vi "Snap To Grid.vi"(0 "Display State In":T1, 7 "Point In":T2) -> (8 "Point Out":cluster{"Horizontal":dbl, "Vertical":dbl})   [LabVIEW 2015, in "FSM Editor.xctl"]
uses:
  FSM Editor.xctl
  <vilib>/Utility/miscctls.llb/LVPoint32TypeDef.ctl
  State.vi
  Classes/FSM.Port/FSM.Port.lvclass
  Drag Mode.ctl
  Events.ctl
  NodeAdded.ctl
  NodeSelected.ctl
  EdgeEventData.ctl
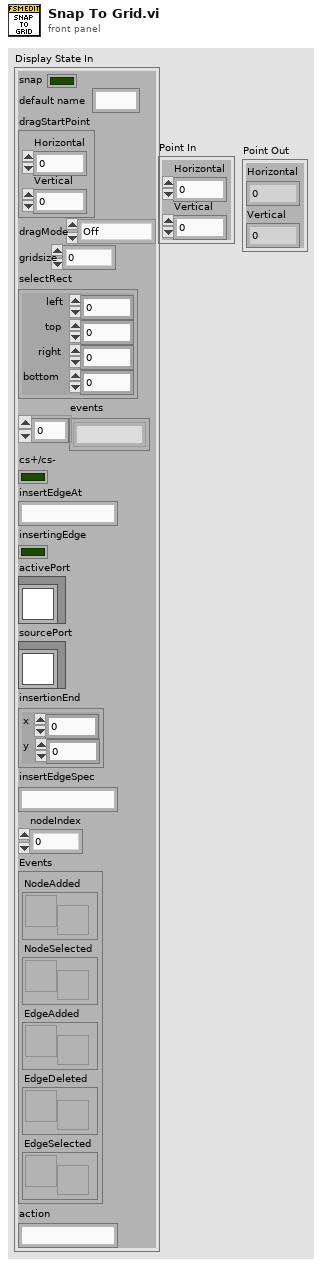
[diagram p1: front panel]
types:
  T1 = typedef "FSM Editor.xctl/State.vi" = cluster{"snap":bool, "default name":string, "dragStartPoint":T2, "dragMode":T3, "gridsize":dbl, "selectRect":cluster{"left":i16, "top":i16, "right":i16, "bottom":i16}, "events":string[], "cs+/cs-":bool, "insertEdgeAt":string, "insertingEdge":bool, "activePort":refnum<class "FSM.Port.lvclass">, "sourcePort":refnum<class "FSM.Port.lvclass">, "insertionEnd":cluster{"x":i16, "y":i16}, "insertEdgeSpec":string, "nodeIndex":i32, "Events":T4, "action":string}
  T2 = typedef "LVPoint32TypeDef.ctl" = cluster{"Horizontal":i32, "Vertical":i32}
  T3 = typedef "Drag Mode.ctl" = enum16{"Off", "NodePending", "Nodes", "Pan", "Select", "EdgeInsertion", "EdgePoint", "EdgeLabel"}
  T4 = typedef "FSM Editor.xctl/Events.ctl" = cluster{"NodeAdded":refnum<user-event>, "NodeSelected":refnum<user-event>, "EdgeAdded":refnum<user-event>, "EdgeDeleted":refnum<user-event>, "EdgeSelected":refnum<user-event>}
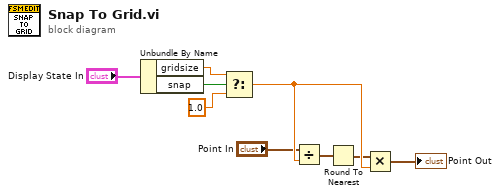
[diagram p0: block diagram]
diagram:
  n1 = Unbundle By Name("Display State In") -> ("gridsize"=w4:dbl, "snap"=w1:bool)
  n2 = Select(t=w4, s=w1, f=1.0) -> (s? t:f=w8:dbl)
  n3 = Divide(x="Point In", y=w8) -> (x/y=w6:cluster{"Horizontal":dbl, "Vertical":dbl})
  n4 = Round To Nearest(number=w6) -> (nearest integer value=w5:cluster{"Horizontal":dbl, "Vertical":dbl})
  n5 = Multiply(x=w5, y=w8) -> (x*y=→"Point Out":cluster{"Horizontal":dbl, "Vertical":dbl})
